vi "RectanglesCalculate.vi"(0 "Max":refnum<vi>) -> (5 "Array":dbl[][](array[numeric]))   [LabVIEW 2009]
uses:
  <vilib>/Analysis/NI_AALBase.lvlib
panel:
  in  "Max 2":cluster{"Max1":dbl[], dbl[]}[](graph)
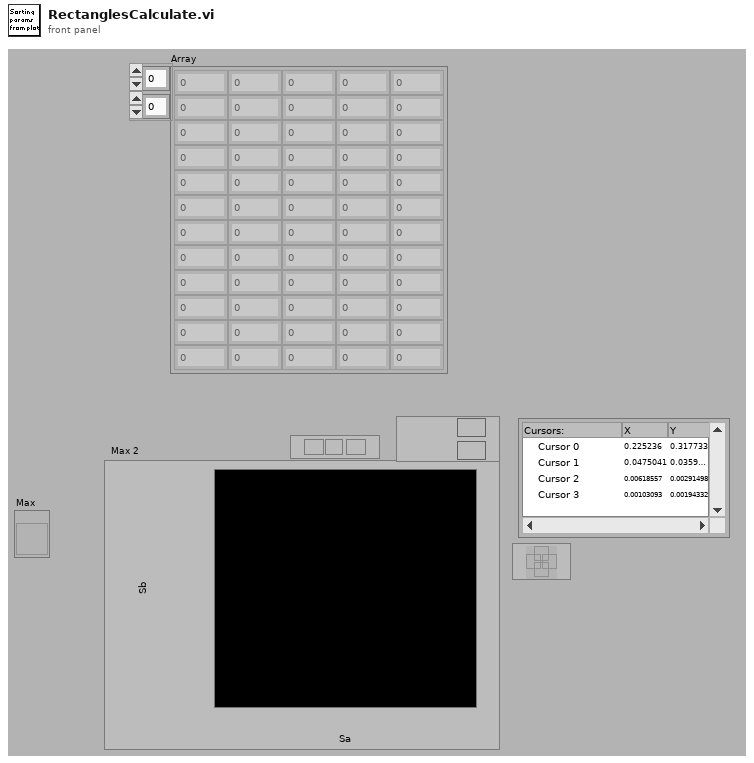
[diagram p1: front panel]
types:
  T1 = typedef "LVPointDoubleTypeDef.ctl" = cluster{"Cursor X":dbl, "Cursor Y":dbl}
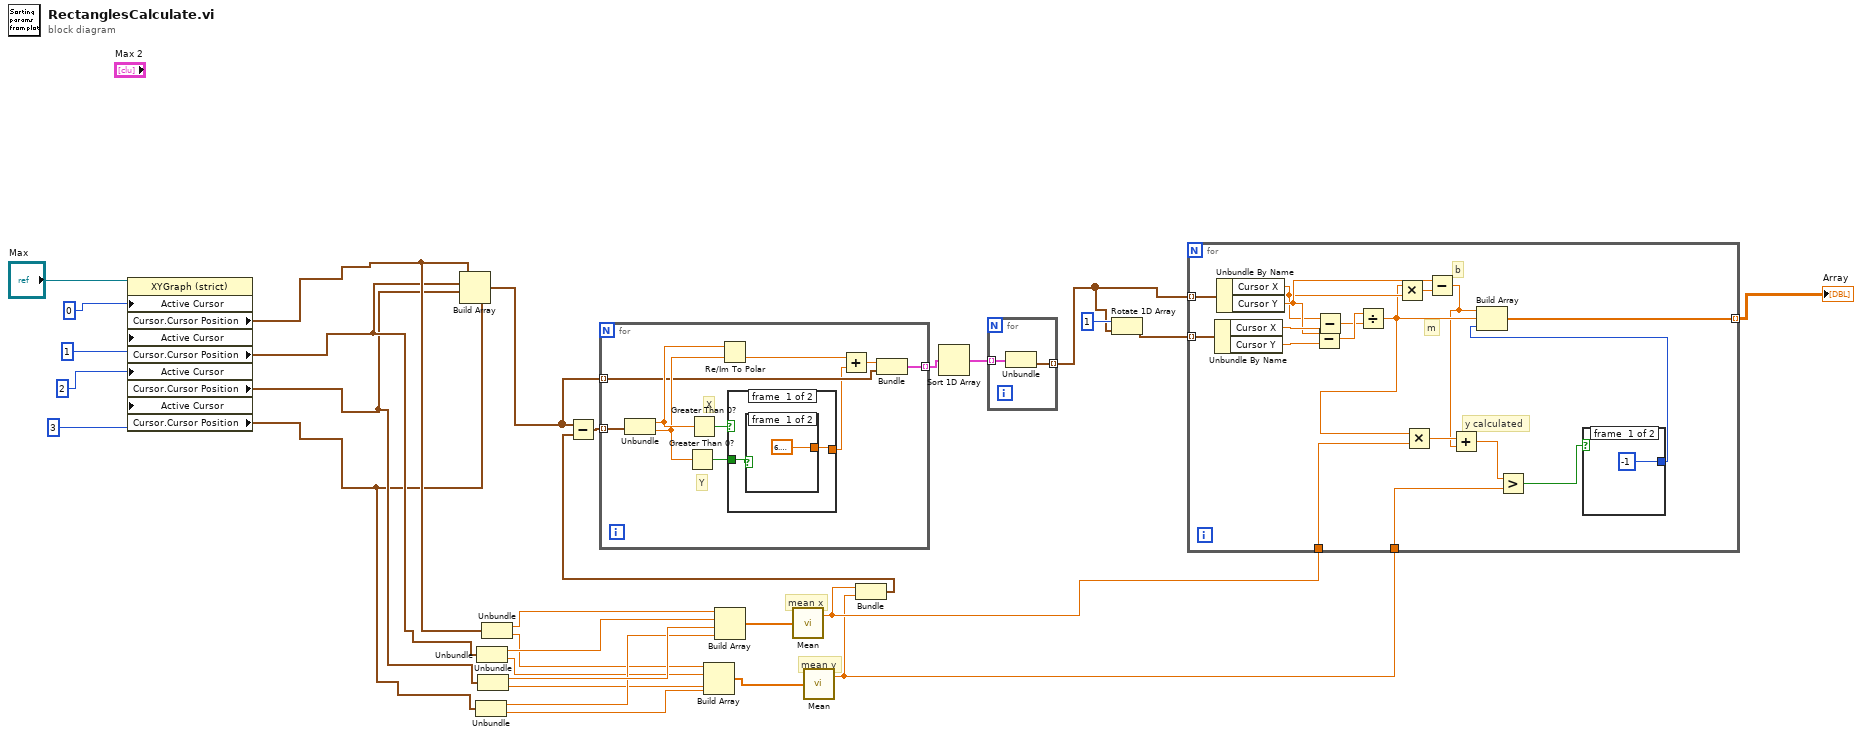
[diagram p0: block diagram]
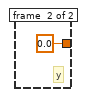
[diagram p2: hidden frame]
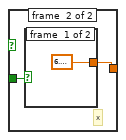
[diagram p3: hidden frame]
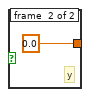
[diagram p4: hidden frame]
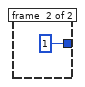
[diagram p5: hidden frame]
diagram:
  # "mean y"
  # "mean x"
  n1 = property on="Property Node" class="XYGraph (strict)"(reference="Max", "Active Cursor"=0, "Active Cursor"=1, "Active Cursor"=2, "Active Cursor"=3) -> ("Cursor.Cursor Position"=w28:T1, "Cursor.Cursor Position"=w27:T1, "Cursor.Cursor Position"=w26:T1, "Cursor.Cursor Position"=w25:T1)  [unwired: 1 in, 2 out]
  n2 = Build Array(w28, w27, w26, w25) -> (w6:T1[])
  n3 = Unbundle(w25) -> ("Cursor X"=w21:dbl, "Cursor Y"=w16:dbl)
  n4 = Unbundle(w27) -> ("Cursor X"=w23:dbl, "Cursor Y"=w18:dbl)
  n5 = Unbundle(w26) -> ("Cursor X"=w22:dbl, "Cursor Y"=w17:dbl)
  n6 = Unbundle(w28) -> ("Cursor X"=w24:dbl, "Cursor Y"=w19:dbl)
  n7 = Build Array(w19, w18, w17, w16) -> (w15:dbl[])
  n8 = Build Array(w24, w23, w22, w21) -> (w20:dbl[])
  n9 = call <vilib>:"Mean.vi"("X"=w20) -> ("mean"=w13:dbl)  [unwired: 1 out]
  n10 = call <vilib>:"Mean.vi"("X"=w15) -> ("mean"=w12:dbl)  [unwired: 1 out]
  n11 = Bundle("mean"=w13, "mean"=w12) -> (w11:cluster{"mean":dbl, "mean":dbl})  [unwired: 1 in]
  n12 = Subtract(x=w6, y=w11) -> (x-y=w10:T1[])
  n13 = for {
    tunnel: w10 -> [w35] mode=indexing
    tunnel: [w34] -> w9 mode=indexing
    tunnel: w6 -> [w33] mode=indexing
    # "Y"
    # "X"
    n14 = Unbundle(w35) -> ("Cursor X"=w39:dbl, "Cursor Y"=w37:dbl)
    n15 = Greater Than 0?(x=w37) -> (x > 0?=w38:bool)
    n16 = Greater Than 0?(x=w39) -> (x > 0?=w40:bool)
    n17 = Re/Im To Polar(2:w37, 3:w39) -> (0:w31:dbl)  [unwired: 1 out]
    n18 = case shown="False" w40 {
      tunnel: w38 -> [w42 w46]
      tunnel: [w41 w45] -> w32
      frame #0 {
        n19 = case shown="False" w42 {
          tunnel: [6.283185307179586 0.0] -> w41
          frame #0 {
          }
          frame #1 {
            # "y"
          }
        }
      }
      frame #1 {
        # "x"
        n20 = case shown="False" w46 {
          tunnel: [6.283185307179586 0.0 ("Cursor Y")] -> w45
          frame #0 {
          }
          frame #1 {
            # "y"
          }
        }
      }
    }
    n21 = Add(x=w31, y=w32) -> (x+y=w36:dbl)
    n22 = Bundle(w36, "Cursor.Cursor Position"=w33) -> (w34:cluster{dbl, "Cursor.Cursor Position":T1})  [unwired: 1 in]
  }
  n23 = Sort 1D Array(array=w9) -> (sorted array=w8:cluster{dbl, "Cursor.Cursor Position":T1}[])
  n24 = for {
    tunnel: w8 -> [w50] mode=indexing
    tunnel: [w49] -> w7 mode=indexing
    n25 = Unbundle(w50) -> ("Cursor.Cursor Position"=w49:T1)  [unwired: 1 out]
  }
  n26 = Rotate 1D Array(1:w7, 2:1) -> (0:w30:T1[])
  n27 = for {
    tunnel: w7 -> [w68] mode=indexing
    tunnel: w30 -> [w67] mode=indexing
    tunnel: [w59] -> w14 mode=indexing
    tunnel: w13 -> [w57]
    tunnel: w12 -> [w51]
    # "y calculated"
    # "m"
    # "b"
    n28 = Unbundle By Name(w67) -> ("Cursor X"=w66:dbl, "Cursor Y"=w65:dbl)
    n29 = Unbundle By Name(w68) -> ("Cursor X"=w61:dbl, "Cursor Y"=w62:dbl)
    n30 = Subtract(x=w62, y=w65) -> (x-y=w64:dbl)
    n31 = Subtract(x=w61, y=w66) -> (x-y=w63:dbl)
    n32 = Divide(x=w64, y=w63) -> (x/y=w58:dbl)
    n33 = Multiply(x=w58, y=w61) -> (x*y=w60:dbl)
    n34 = Multiply(x=w58, y=w57) -> (x*y=w56:dbl)
    n35 = Subtract(x=w62, y=w60) -> (x-y=w55:dbl)
    n36 = Add(x=w56, y=w55) -> (x+y=w52:dbl)
    n37 = Greater?(x=w52, y=w51) -> (0:w54:bool)
    n38 = case shown="True" w54 {
      tunnel: [-1 1] -> w53
      frame #0 {
      }
      frame #1 {
      }
    }
    n39 = Build Array(w55, w58, w53) -> (w59:dbl[])
  }
  "Array" <- w14
